vi "Reverse (single).vi"(8 "error in (no error)":errorcluster, 11 "XY-data":cluster{"X-array":dbl[], "Y-array":dbl[]}) -> (0 "error out":errorcluster, 3 "Reversed XY-data out":cluster{"X-array":dbl[], "Y-array":dbl[]} {"Y-array" format="%.2p"; "X-array" format="%.2p"})   [LabVIEW 2016, in "xy_utilities.lvlib"]
doc: "Reverse both x and y arrays.\n\nWire data to the data input to determine the polymorphic instance to use or manually select the instance."
uses:
  xy_utilities.lvlib
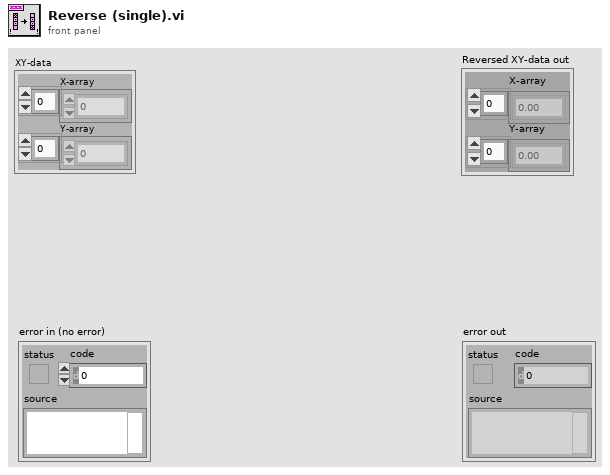
[diagram p1: front panel]
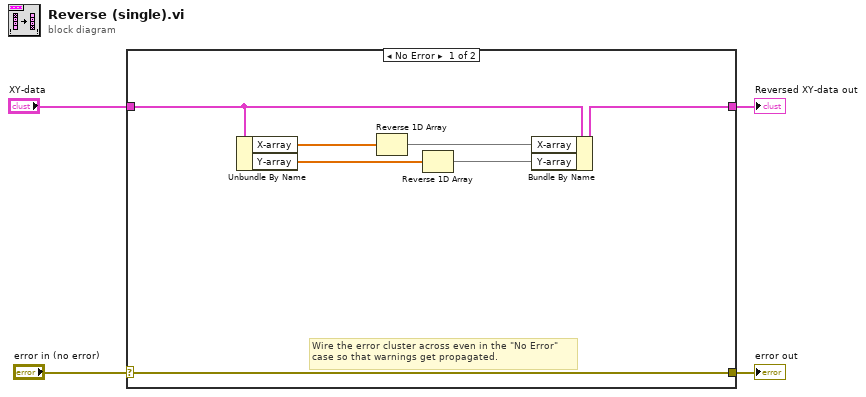
[diagram p0: block diagram]
diagram:
  n1 = case shown="No Error" "error in (no error)" {
    selector: "error in (no error)" -> [w11 w13]
    tunnel: [w11 w13] -> w3
    tunnel: "XY-data" -> [w10 w12]
    tunnel: [w9 w12] -> w1
    frame No Error {
      # "Wire the error cluster across even in the \"No Error\"\ncase so that warnings get propagated."
      n2 = Unbundle By Name(w10) -> ("X-array"=w7:dbl[], "Y-array"=w5:dbl[])
      n3 = Reverse 1D Array(array=w7) -> (reversed array=w8:dbl[])
      n4 = Reverse 1D Array(array=w5) -> (reversed array=w6:dbl[])
      n5 = Bundle By Name(cluster=w10, "X-array"=w8, "Y-array"=w6) -> (w9:cluster{"X-array":dbl[], "Y-array":dbl[]})
    }
    frame Error {
    }
  }
  "error out" <- w3
  "Reversed XY-data out" <- w1
